vi "RSZVB Get Two Port Transmission Coefficients Enabled.vi"(8 "error in (no error)":errorcluster {"code" format="%.0x"}, 11 "VISA session":refnum<visa-resource-name>) -> (0 "error out":errorcluster {"code" format="%.0x"}, 2 "Two-Port Enabled":bool, 3 "dup VISA session":refnum<visa-resource-name>)   [LabVIEW 2011]
doc: "This VI returns the use of two-port transmission coefficients. \n\nRemote-control command(s):\nSOURce<Ch>:POWer<Pt>:CORRection:TCOefficient[:STATe]?"
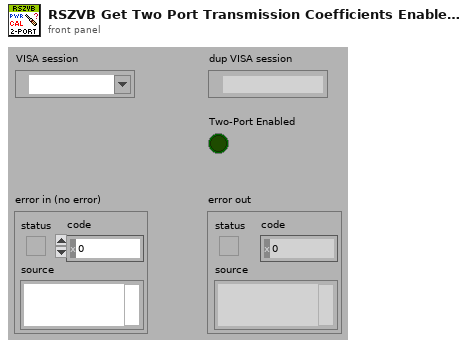
[diagram p1: front panel]
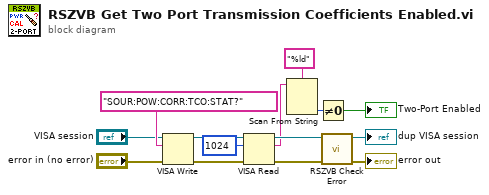
[diagram p0: block diagram]
diagram:
  n1 = VISA Write(VISA resource name="VISA session", write buffer="SOUR:POW:CORR:TCO:STAT?", error in (no error)="error in (no error)") -> (VISA resource name out=w10:refnum<visa-resource-name>, error out=w11:errorcluster)  [unwired: 1 out]
  n2 = VISA Read(VISA resource name=w10, byte count=u32 1024, error in (no error)=w11) -> (VISA resource name out=w12:refnum<visa-resource-name>, read buffer=w4:string, error out=w13:errorcluster)  [unwired: 1 out]
  n3 = Scan From String(format string="%ld", input string=w4) -> (output 1=w2:i32)  [unwired: 3 in, 3 out]
  n4 = Not Equal To 0?(x=w2) -> (x != 0?=→"Two-Port Enabled":bool)
  n5 = call "RSZVB Check Error.vi"("error in (no error)"=w13, "VISA session"=w12) -> ("error out"=→"error out":errorcluster, "dup VISA session"=→"dup VISA session":refnum<visa-resource-name>)  [unwired: 8 in]
